vi "DisplayDeviceTable.vi"(3 "error in (no error)":errorcluster, 4 "Device Table In":refnum<k24>, 5 "Output Refnum In":refnum<vi>) -> (0 "error out":errorcluster, 1 "Device Table Out":refnum<k24>, 2 "Output Refnum Out":refnum<vi>)   [LabVIEW 2009]
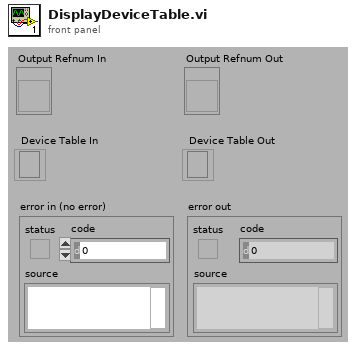
[diagram p1: front panel]
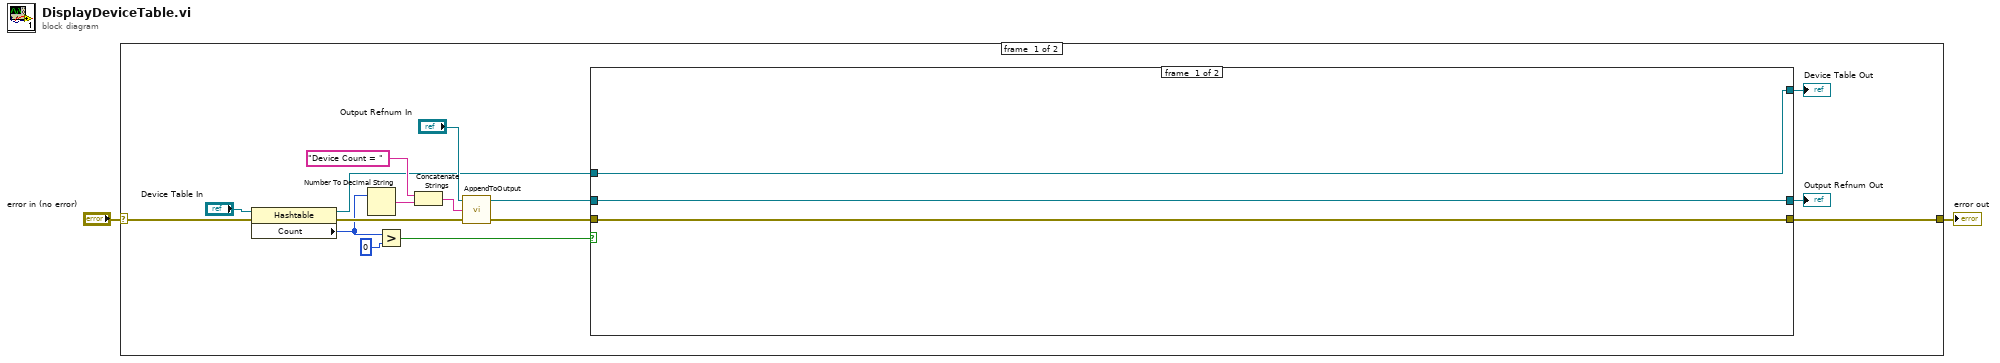
[diagram p0: block diagram]
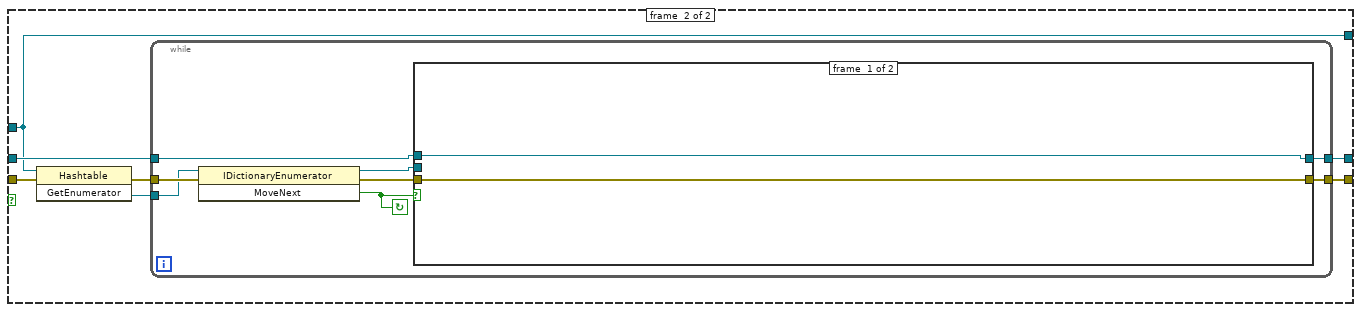
[diagram p2: hidden frame]
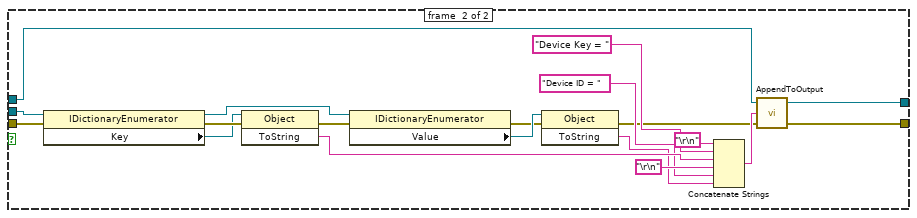
[diagram p3: hidden frame]
diagram:
  n1 = case shown="No Error" "error in (no error)" {
    selector: "error in (no error)" -> [w3 w58]
    tunnel: [w5 w58] -> w2
    frame #0 {
      n2 = property class="Hashtable"(reference="Device Table In", error in=w3) -> (reference out=w11:refnum<k24>, error out=w13:errorcluster, "Count"=w10:i32)
      n3 = Number To Decimal String(number=w10) -> (decimal integer string=w15:string)  [unwired: 1 in]
      n4 = Greater?(x=w10, y=0) -> (0:w8:bool)
      n5 = Concatenate Strings("Device Count = ", w15) -> (w17:string)
      n6 = call "AppendToOutput.vi"("error in"=w13, "Input String"=w17, "Output Refnum In"="Output Refnum In") -> ("error out"=w12:errorcluster, "Output Refnum Out"=w7:refnum<vi>)  [unwired: 1 in]
      n7 = case shown="True" w8 {
        tunnel: w12 -> [w21 w28]
        tunnel: w11 -> [w20 w22]
        tunnel: w7 -> [w19 w25]
        tunnel: [w19 w24] -> w6
        tunnel: [w21 w23] -> w5
        tunnel: [w20 w22] -> w4
        frame #0 {
        }
        frame #1 {
          n8 = invoke class="Hashtable" method="GetEnumerator"(reference=w22, error in=w28) -> (error out=w27:errorcluster, "GetEnumerator"=w26:refnum<k24>)  [unwired: 1 in, 1 out]
          n9 = while {
            tunnel: w27 -> [w36]
            tunnel: w26 -> [w35]
            tunnel: w25 -> [w31]
            tunnel: [w30] -> w24
            tunnel: [w29] -> w23
            stop <- w32 continue-if-true
            n10 = invoke class="IDictionaryEnumerator" method="MoveNext"(reference=w35, error in=w36) -> (reference out=w34:refnum<k24>, error out=w33:errorcluster, "MoveNext"=w32:bool)  [unwired: 1 in]
            n11 = case shown="True" w32 {
              tunnel: w34 -> [_ w57]
              tunnel: w33 -> [w38 w56]
              tunnel: w31 -> [w37 w42]
              tunnel: [w37 w40] -> w30
              tunnel: [w38 w39] -> w29
              frame #0 {
              }
              frame #1 {
                n12 = property class="IDictionaryEnumerator"(reference=w57, error in=w56) -> (reference out=w48:refnum<k24>, error out=w55:errorcluster, "Key"=w54:refnum<k24>)
                n13 = invoke class="Object" method="ToString"(reference=w54, error in=w55) -> (error out=w47:errorcluster, "ToString"=w52:string)  [unwired: 1 in, 1 out]
                n14 = property class="IDictionaryEnumerator"(reference=w48, error in=w47) -> (error out=w45:errorcluster, "Value"=w46:refnum<k24>)  [unwired: 1 out]
                n15 = invoke class="Object" method="ToString"(reference=w46, error in=w45) -> (error out=w41:errorcluster, "ToString"=w44:string)  [unwired: 1 in, 1 out]
                n16 = Concatenate Strings("\r\n", "Device Key = ", w52, "\r\n", "Device ID = ", w44) -> (w43:string)
                n17 = call "AppendToOutput.vi"("error in"=w41, "Input String"=w43, "Output Refnum In"=w42) -> ("error out"=w39:errorcluster, "Output Refnum Out"=w40:refnum<vi>)  [unwired: 1 in]
              }
            }
          }
        }
      }
      "Device Table Out" <- w4
      "Output Refnum Out" <- w6
    }
    frame #1 {
    }
  }
  "error out" <- w2
